vi "UI - Top VI.vi"(8 "error in":errorcluster) -> (0 "error out":errorcluster)   [LabVIEW 2024, in "User Interface.lvlib"]
uses:
  User Interface.lvlib
  Support/General Type Defs/Device Data.ctl
  Support/General Type Defs/Device OS.ctl
  Support/General Type Defs/Global Data.vi
  UI Queue - Dequeue.vi
  Session Scanner/Scanner Queue - Enqueue.vi
  UI Queue - Enqueue.vi
  Data Base/DataBase Queue - Enqueue.vi
  UI Queue - Destroy.vi
  Session Scanner/Session Scanner.lvlib
  Support/General Type Defs/General Type Defs.lvlib
  Data Base/Data Base.lvlib
panel:
  out "Message":string
  in  "Tab Control":enum32{"Scanner", "Devices List"}(tab)
  out "In Use?":bool
  in  "Devices":string(combo)="NEW DEVICE"
  in  "Device Data":T1
  in  "Search":bool
  out "Sessions":string[][](table)
  out "Devices Table":string[][](table)
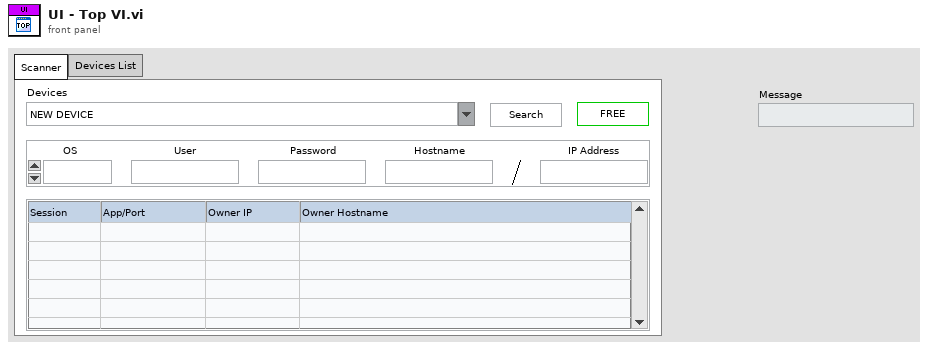
[diagram p1: front panel]
types:
  T1 = typedef "General Type Defs.lvlib/Device Data.ctl" = cluster{"OS":T2, "User":string, "Password":string, "Hostname":string, "IP Address":string}
  T2 = typedef "General Type Defs.lvlib/Device OS.ctl" = enum16{"Windows", "Linux"}
  T3 = enum8{"Enabled", "Disabled", "Disabled and Grayed Out"}
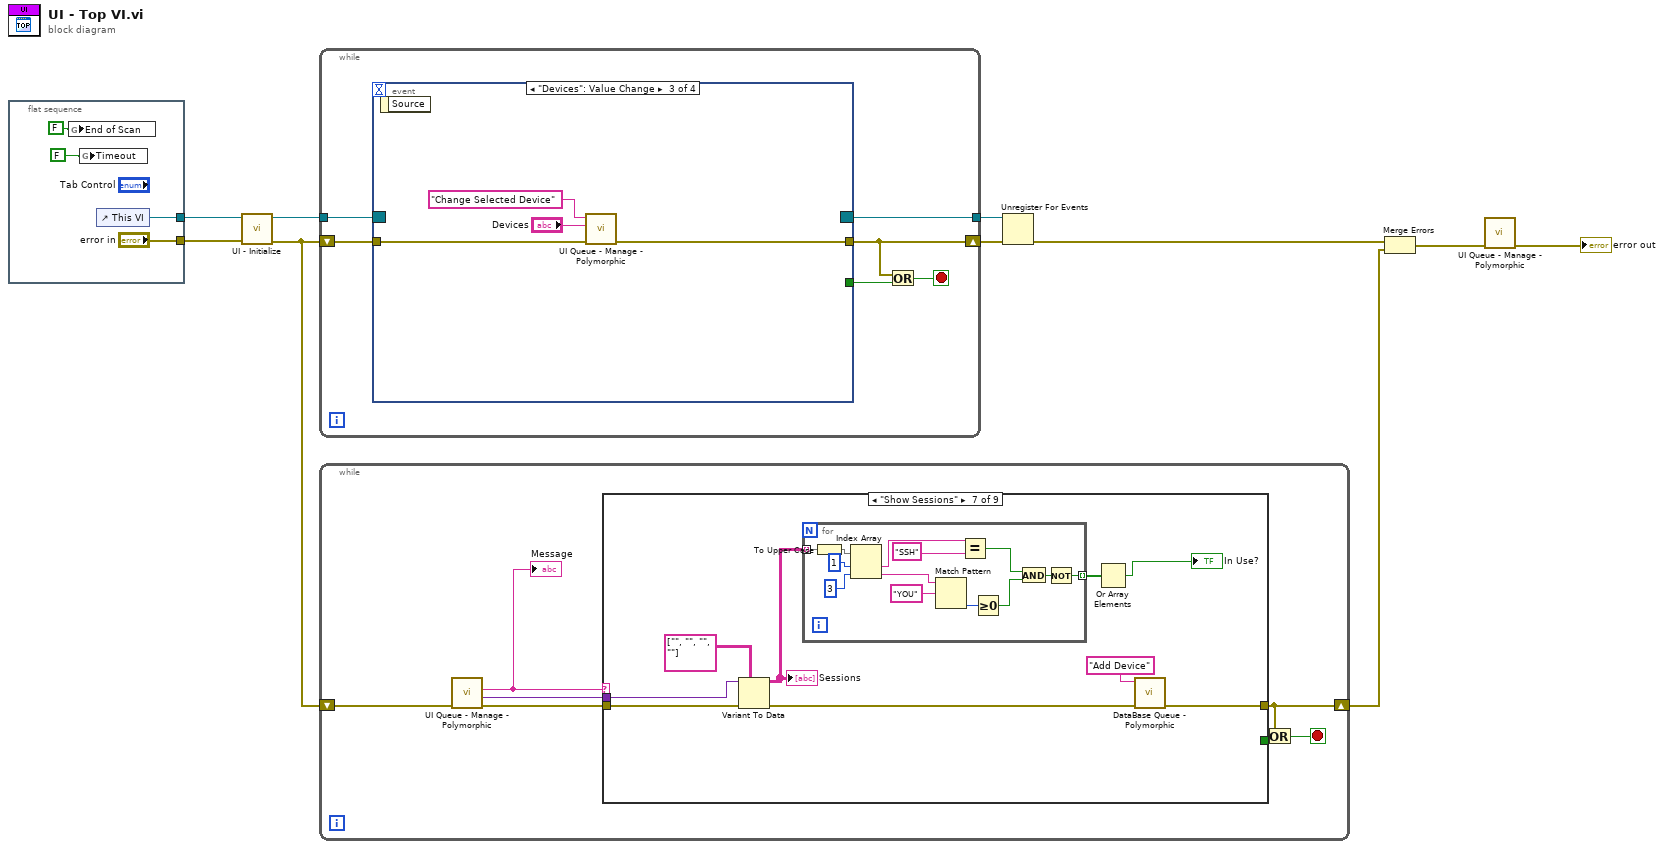
[diagram p0: block diagram]
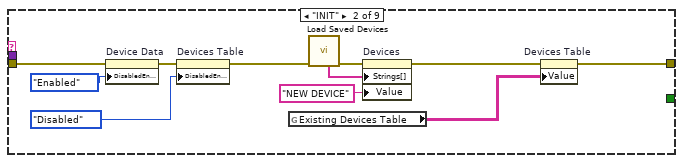
[diagram p3: hidden frame]
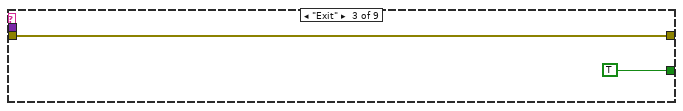
[diagram p4: hidden frame]
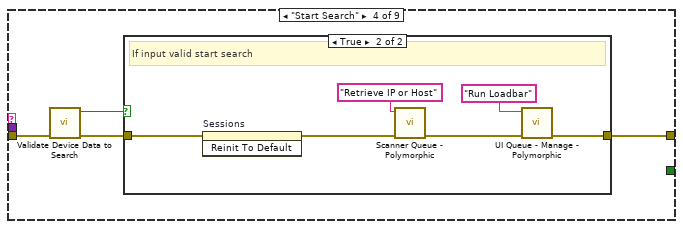
[diagram p5: hidden frame]
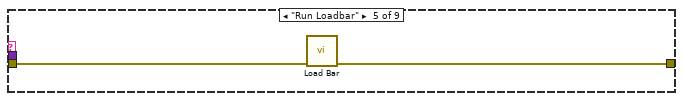
[diagram p7: hidden frame]
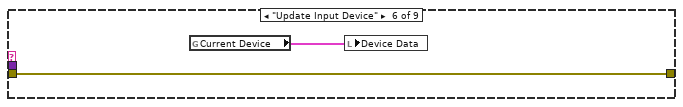
[diagram p8: hidden frame]
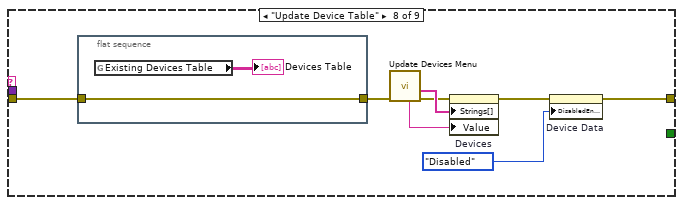
[diagram p9: hidden frame]
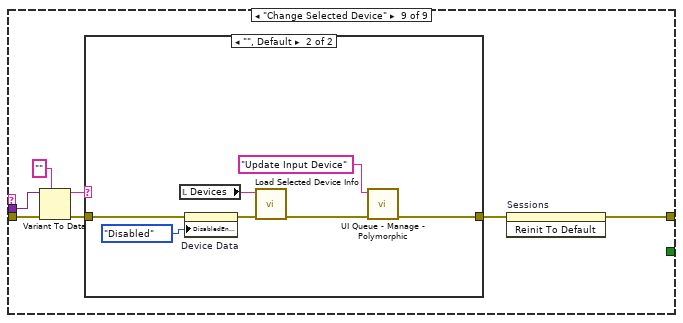
[diagram p10: hidden frame]
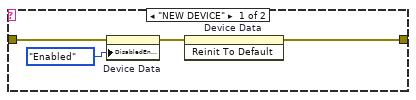
[diagram p11: hidden frame]
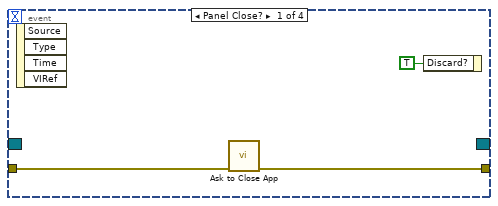
[diagram p12: hidden frame]
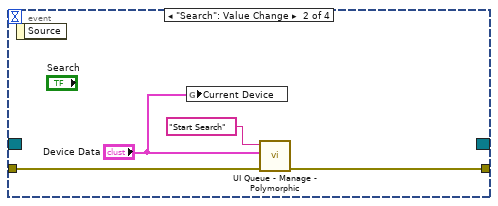
[diagram p13: hidden frame]
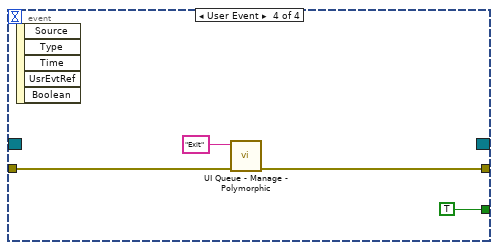
[diagram p14: hidden frame]
diagram:
  n1 = flat-sequence {
    tunnel: [w14] -> w10
    tunnel: ["error in"] -> w1
    frame #0 {
      n2 = global write "Global Data.vi" "End of Scan"(FALSE ("End of Scan")) -> ()
      n3 = global write "Global Data.vi" "Timeout"(FALSE ("Timeout")) -> ()
      n4 = control-ref of="This VI"() -> (w14:refnum<vi>)
    }
  }
  n5 = call "UI - Initialize.vi"("error in (no error)"=w1, "VI In"=w10) -> ("error out"=w6:errorcluster, "Event Registration Out"=w9:refnum<event-registration>)  [unwired: 8 in]
  n6 = while {
    tunnel: w9 -> [w20]
    shift-right: [w15] -> w8
    shift-left: w6 -> [w19]
    tunnel: [w18] -> w7
    stop <- w16 stop-if-true
    n7 = event shown="[2] \"Devices\": Value Change" {
      selector: w20 -> [_ _ _ _]
      dyn-events: [_ _ _ _] -> w18
      timeout: _ -> [_ _ _ _]
      tunnel: w19 -> [w23 w27 w31 w34]
      tunnel: [w22 w26 w30 w33] -> w15
      tunnel: [_ _ _ TRUE] -> w17
      event Panel Close? {
        n8 = event-data() -> ()  [unwired: 1 in, 4 out]
        n9 = call "Ask to Close App.vi"("error in"=w23) -> ("error out"=w22:errorcluster)  [unwired: 10 in]
        n10 = event-data("Discard?"=TRUE) -> ()  [unwired: 1 in, 1 out]
      }
      event "Search": Value Change {
        n11 = event-data() -> ()  [unwired: 1 in, 1 out]
        n12 = global write "Global Data.vi" "Current Device"("Device Data") -> ()
        n13 = call-poly "UI Queue - Manage - Polymorphic.vi"("error in"=w27, "Value"="Device Data", "Message"="Start Search") -> ("error out"=w26:errorcluster)  [unwired: 8 in]
      }
      event "Devices": Value Change {
        n14 = event-data() -> ()  [unwired: 1 in, 1 out]
        n15 = call-poly "UI Queue - Manage - Polymorphic.vi"("error in"=w31, "Value"="Devices", "Message"="Change Selected Device") -> ("error out"=w30:errorcluster)  [unwired: 8 in]
      }
      event User Event {
        n16 = event-data() -> ()  [unwired: 1 in, 5 out]
        n17 = call-poly "UI Queue - Manage - Polymorphic.vi"("error in"=w34, "Message"="Exit") -> ("error out"=w33:errorcluster)  [unwired: 9 in]
      }
    }
    n18 = Or(x=w15, y=w17) -> (x .or. y?=w16:bool)
  }
  n19 = while {
    shift-right: [w37] -> w4
    shift-left: w6 -> [w42]
    stop <- w38 stop-if-true
    n20 = call-poly "UI Queue - Manage - Polymorphic.vi"("error in"=w42) -> ("error out"=w40:errorcluster, "Message Data"=w41:variant, "Message"=w36:string)  [unwired: 8 in]
    "Message" <- w36
    n21 = case shown="\"Show Sessions\"" w36 {
      tunnel: w41 -> [_ _ _ _ _ _ w79 _ w109]
      tunnel: w40 -> [w43 w54 w56 w60 w69 w71 w80 w101 w110]
      tunnel: [w43 w45 w56 w57 w68 w71 w76 w95 w104] -> w37
      tunnel: [_ _ TRUE _ _ _ _ _ _] -> w39
      frame "IDLE", Default {
      }
      frame "INIT" {
        n22 = property on="Device Data" class="Clust (strict)"(error in=w54, "DisabledEnum"=T3."Enabled" ("Disabled")) -> (error out=w52:errorcluster)  [unwired: 1 in, 1 out]
        n23 = property on="Devices Table" class="Tbl (strict)"(error in=w52, "DisabledEnum"=T3."Disabled" ("Disabled")) -> (error out=w48:errorcluster)  [unwired: 1 in, 1 out]
        n24 = global read "Global Data.vi" "Existing Devices Table"() -> (w44:string[][])
        n25 = call "Load Saved Devices.vi"("error in"=w48) -> ("error out"=w47:errorcluster, "Menu Devices"=w49:string[])  [unwired: 9 in]
        n26 = property on="Devices" class="CmbBox"(error in=w47, "Strings[]"=w49, "Value"="NEW DEVICE") -> (error out=w46:errorcluster)  [unwired: 1 in, 1 out]
        n27 = property on="Devices Table" class="Tbl (strict)"(error in=w46, "Value"=w44) -> (error out=w45:errorcluster)  [unwired: 1 in, 1 out]
      }
      frame "Exit" {
      }
      frame "Start Search" {
        n28 = call "Validate Device Data to Search.vi"("error in (no error)"=w60) -> ("error out"=w58:errorcluster, "Valid Device?"=w59:bool)  [unwired: 9 in]
        n29 = case shown="True" w59 {
          tunnel: w58 -> [w61 w63]
          tunnel: [w61 w65] -> w57
          frame False {
          }
          frame True {
            # "If input valid start search"
            n30 = invoke on="Sessions" class="Tbl (strict)" method="Reinit To Default"(error in=w63) -> (error out=w62:errorcluster)  [unwired: 2 in, 2 out]
            n31 = call-poly "Scanner Queue - Polymorphic.vi"("error in"=w62, "Message"="Retrieve IP or Host") -> ("error out"=w66:errorcluster)  [unwired: 9 in]
            n32 = call-poly "UI Queue - Manage - Polymorphic.vi"("error in"=w66, "Message"="Run Loadbar") -> ("error out"=w65:errorcluster)  [unwired: 9 in]
          }
        }
      }
      frame "Run Loadbar" {
        n33 = call "Load Bar.vi"("error in"=w69) -> ("error out"=w68:errorcluster)  [unwired: 10 in]
      }
      frame "Update Input Device" {
        n34 = global read "Global Data.vi" "Current Device"() -> (w70:T1)
        n35 = local write "Device Data"(w70) -> ()
      }
      frame "Show Sessions" {
        n36 = Variant To Data(error in=w80, type=string[][] [["", "", "", ""]] ("Sessions"), Variant=w79) -> (data=w74:string[][], error out=w77:errorcluster)
        "Sessions" <- w74
        n37 = for {
          tunnel: w74 -> [w93] mode=indexing
          tunnel: [w81] -> w73 mode=indexing
          n38 = To Upper Case(1:w93) -> (0:w90:string[])
          n39 = Index Array(array=w90, index #1=1 ("index"), index #2=3 ("index")) -> (element #1=w86:string, element #2=w88:string)
          n40 = Match Pattern(string=w88, regular expression="YOU") -> (offset past match=w87:i32)  [unwired: 1 in, 3 out]
          n41 = Equal?(x=w86, y="SSH" ("regular expression")) -> (x = y?=w84:bool)
          n42 = Greater Or Equal To 0?(x=w87) -> (x >= 0?=w83:bool)
          n43 = And(x=w84, y=w83) -> (x .and. y?=w82:bool)
          n44 = Not(x=w82) -> (.not. x?=w81:bool)
        }
        n45 = Or Array Elements(Boolean array=w73) -> (logical OR=→"In Use?":bool)
        n46 = call-poly "DataBase Queue - Polymorphic.vi"("error in"=w77, "Message"="Add Device") -> ("error out"=w76:errorcluster)  [unwired: 9 in]
      }
      frame "Update Device Table" {
        n47 = flat-sequence {
          tunnel: w101 -> [w102]
          tunnel: [w102] -> w100
          frame #0 {
            n48 = global read "Global Data.vi" "Existing Devices Table"() -> (→"Devices Table":string[][])
          }
        }
        n49 = call "Update Devices Menu.vi"("error in"=w100) -> ("error out"=w98:errorcluster, "New Menu"=w99:string[], "Device for Search"=w97:string)  [unwired: 8 in]
        n50 = property on="Devices" class="CmbBox"(error in=w98, "Strings[]"=w99, "Value"=w97) -> (error out=w96:errorcluster)  [unwired: 1 in, 1 out]
        n51 = property on="Device Data" class="Clust (strict)"(error in=w96, "DisabledEnum"=T3."Disabled" ("Disabled")) -> (error out=w95:errorcluster)  [unwired: 1 in, 1 out]
      }
      frame "Change Selected Device" {
        n52 = Variant To Data(error in=w110, type="" ("Message"), Variant=w109) -> (data=w106:string, error out=w107:errorcluster)
        n53 = case shown="\"\", Default" w106 {
          tunnel: w107 -> [w113 w117]
          tunnel: [w111 w120] -> w105
          frame "NEW DEVICE" {
            n54 = property on="Device Data" class="Clust (strict)"(error in=w113, "DisabledEnum"=T3."Enabled" ("Disabled")) -> (error out=w112:errorcluster)  [unwired: 1 in, 1 out]
            n55 = invoke on="Device Data" class="Clust (strict)" method="Reinit To Default"(error in=w112) -> (error out=w111:errorcluster)  [unwired: 2 in, 2 out]
          }
          frame "", Default {
            n56 = local read "Devices"() -> (w118:string)
            n57 = property on="Device Data" class="Clust (strict)"(error in=w117, "DisabledEnum"=T3."Disabled" ("Disabled")) -> (error out=w116:errorcluster)  [unwired: 1 in, 1 out]
            n58 = call "Load Selected Device Info.vi"("error in"=w116, "Selected Device"=w118) -> ("error out"=w119:errorcluster)  [unwired: 9 in]
            n59 = call-poly "UI Queue - Manage - Polymorphic.vi"("error in"=w119, "Message"="Update Input Device") -> ("error out"=w120:errorcluster)  [unwired: 9 in]
          }
        }
        n60 = invoke on="Sessions" class="Tbl (strict)" method="Reinit To Default"(error in=w105) -> (error out=w104:errorcluster)  [unwired: 2 in, 2 out]
      }
    }
    n61 = Or(x=w37, y=w39) -> (x .or. y?=w38:bool)
  }
  n62 = Unregister For Events(event registration refnum=w7, error in=w8) -> (error out=w5:errorcluster)
  n63 = Merge Errors(w5, w4) -> (w3:errorcluster)
  n64 = call-poly "UI Queue - Manage - Polymorphic.vi"("error in"=w3) -> ("error out"=→"error out":errorcluster)  [unwired: 10 in]
